vi "IR_SENSOR[1].vi"() -> ()   [LabVIEW 2018]
panel:
  out "count":dbl
  in  "stop":bool
  out ".not. x?":bool
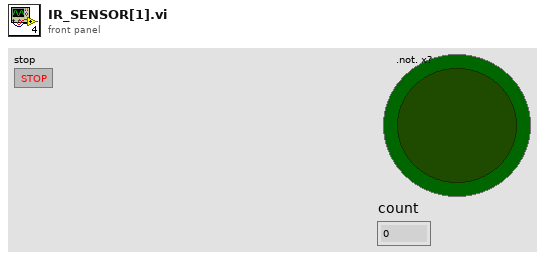
[diagram p1: front panel]
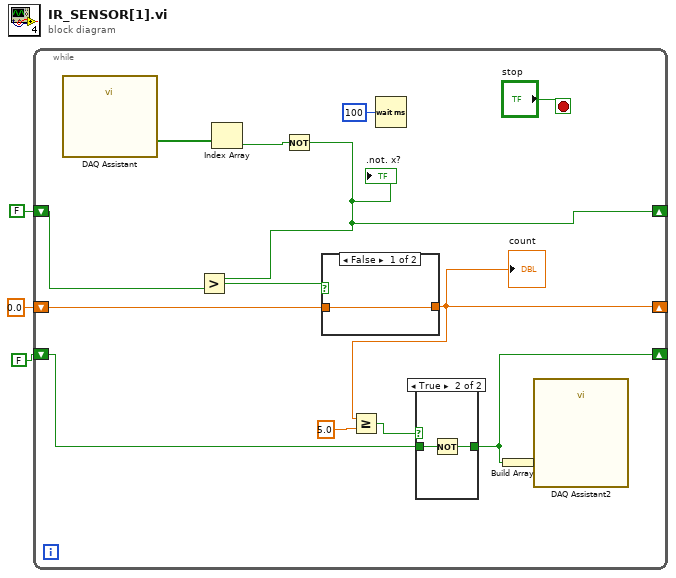
[diagram p0: block diagram]
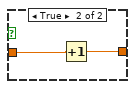
[diagram p3: hidden frame]
diagram:
  n1 = while {
    shift-right: [w13] -> _
    shift-left: FALSE -> [w12]
    shift-right: [w8] -> _
    shift-left: 0.0 -> [w11]
    shift-right: [w5] -> _
    shift-left: FALSE -> [w4]
    stop <- "stop" stop-if-true
    n2 = call "DAQ Assistant"() -> ("data"=w17:bool[])  [unwired: 17 in, 2 out]
    n3 = Index Array(array=w17) -> (element=w16:bool)  [unwired: 1 in]
    n4 = Not(x=w16) -> (.not. x?=w13:bool)
    ".not. x?" <- w13
    n5 = Greater?(x=w13, y=w12) -> (0:w14:bool)
    n6 = case shown="False" w14 {
      tunnel: w11 -> [w21 w22]
      tunnel: [w21 w23] -> w8
      frame False {
      }
      frame True {
        n7 = Increment(x=w22) -> (x+1=w23:dbl)
      }
    }
    "count" <- w8
    n8 = Greater Or Equal?(x=w8, y=5.0) -> (x >= y?=w7:bool)
    n9 = Wait (ms)(milliseconds to wait=u32 100) -> ()  [unwired: 1 out]
    n10 = case shown="True" w7 {
      tunnel: [w18 w20] -> w5
      tunnel: w4 -> [w18 w19]
      frame False {
      }
      frame True {
        n11 = Not(x=w19) -> (.not. x?=w20:bool)
      }
    }
    n12 = Build Array(w5) -> (w6:bool[])
    n13 = call "DAQ Assistant2"("data"=w6) -> ()  [unwired: 17 in, 2 out]
  }
